vi "Convert FITS to IMAQ.vi"() -> ()   [LabVIEW 2023]
uses:
  gfitsio.lvlib
  gfitsio-read-image-subset-i16-2d.vi
  gfitsio-write-key-double.vi
panel:
  in  "file path":path=path "C:/Users/smarlow/Documents/FPA/gain_00014ms_1600x200_0017.fits"
  out "error out":errorcluster
  out "data":i16[][](array[numeric])
  out "Image":T1(plugin-control)
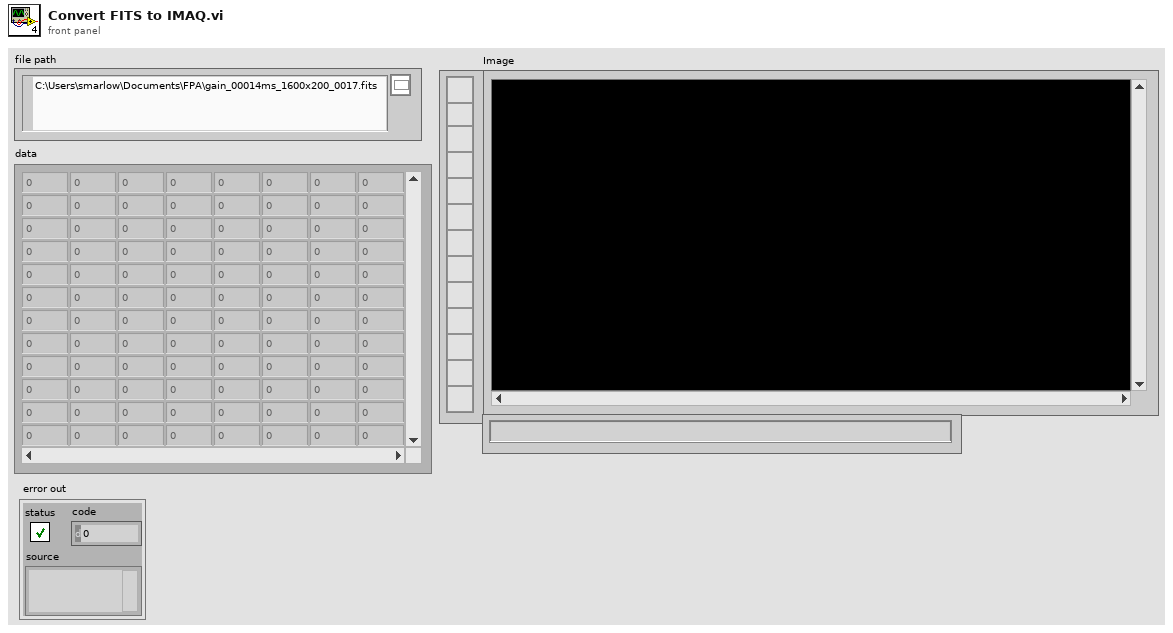
[diagram p1: front panel]
types:
  T1 = typedef "IMAQ Image.ctl" = refnum<image>
  T2 = typedef "Image Type" = u32
  T3 = typedef "gfitsio.lvlib/gfitsio-refnum.ctl" = refnum<k1>
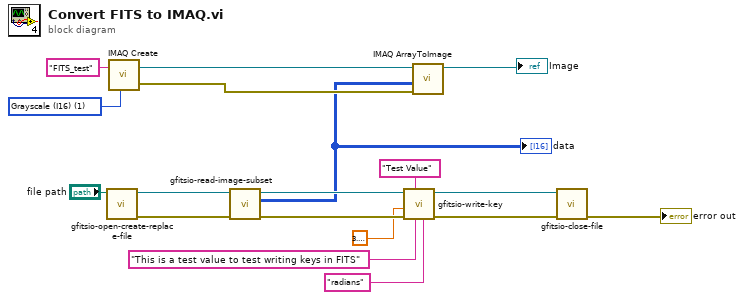
[diagram p0: block diagram]
diagram:
  w13 = T2 1 items=["Grayscale (U8)", "Grayscale (I16)", "Grayscale (SGL)", "Complex (CSG)", "RGB (U32)", "HSL (U32)", "RGB (U64)", "Grayscale (U16)"] ("Image Type")
  n1 = call "gfitsio-open-create-replace-file.vi"("file path (dialog if empty)"="file path") -> ("error out"=w17:errorcluster, "gfits refnum"=w18:T3)  [unwired: 8 in, 1 out]
  n2 = call "IMAQ Create"("Image Name"="FITS_test", "Image Type"=w13) -> ("New Image"=w11:T1, "error out"=w10:errorcluster)  [unwired: 3 in]
  n3 = call-poly "gfitsio-read-image-subset.vi"("error in (no error)"=w17, "gfits refnum"=w18) -> ("error out"=w6:errorcluster, "data"=w8:i16[][], "dup gfits refnum"=w15:T3)  [unwired: 7 in]
  "data" <- w8
  n4 = call-poly "gfitsio-write-key.vi"("units"="radians", "comment"="This is a test value to test writing keys in FITS", "keyname"="Test Value", "error in (no error)"=w6, "value"=3.141592653589793, "gfits refnum"=w15) -> ("error out"=w5:errorcluster, "dup gfits refnum"=w7:T3)  [unwired: 4 in]
  n5 = call "IMAQ ArrayToImage"("error in (no error)"=w10, "Image Pixels (I16)"=w8, "Image"=w11) -> ("Image Out"=→"Image":T1)  [unwired: 7 in, 1 out]
  n6 = call "gfitsio-close-file.vi"("error in (no error)"=w5, "gfits refnum"=w7) -> ("error out"=→"error out":errorcluster)  [unwired: 8 in, 1 out]
